vi "Set FPGA constants.vi"(8 "error in (no error)":errorcluster, 11 "AODAcq in":refnum<class "AODAcq.lvclass">) -> (0 "error out":errorcluster, 3 "AODAcq out":refnum<class "AODAcq.lvclass">)   [LabVIEW 2011, in "AODAcq.lvclass"]
uses:
  AODAcq.lvclass
  FPGA_Control/AODCalibration.ctl
  <vilib>/Utility/error.llb/Error Cluster From Error Code.vi
  Program Files/National Instruments/LabVIEW 2011/Targets/NI/FPGA/StockFPGA_IntfPrivate/ScriptTemplates/StockFPGA_PlugInRead32.vi
  <vilib>/rvi/errors/niLvFpgaAdjustHostInterfaceError.vi
  <vilib>/rvi/interface/nirviReadWriteControl/nirviReadWriteControl.xnode
  FPGA_Control/AODRef.ctl
  FPGA Bitfiles/Acquisition_FPGATarget_AODControl(FPGA)_C1C38267.lvbitx
  FPGA_Control/AOD Control (FPGA).vi
  NiFpgaLv.dll
  <vilib>/FPGAPlugInAG/PXIe-7965R/niLvFpga_Read32_PXIe-7965R.vi
  <vilib>/rvi/interface/nirviReadWriteControl/niFpgaRWControlAccessTimeoutTemplate.vi
panel:
  in  "AOD.BlankSamples":u16=800
  in  "AOD.ThrowawaySamples":u16=1250
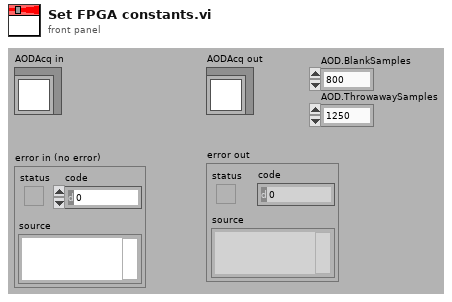
[diagram p1: front panel]
types:
  T1 = typedef "AODCalibration.ctl" = cluster{"XHP ChirpGain":fxp<+/-,16,2>, "YHP ChirpGain":fxp<+/-,16,2>, "XLP ChirpGain":fxp<+/-,16,2>, "YLP ChirpGain":fxp<+/-,16,2>}
  T2 = typedef "AODRef.ctl" = refnum<k20>
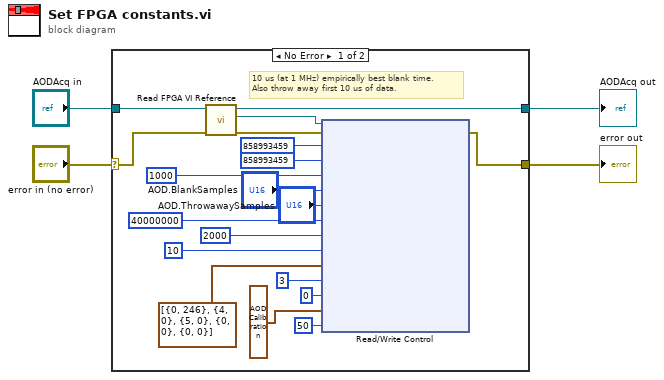
[diagram p0: block diagram]
diagram:
  n1 = case shown="No Error" "error in (no error)" {
    selector: "error in (no error)" -> [w15 w25]
    tunnel: [w14 w25] -> w3
    tunnel: [w22 w24] -> w1
    tunnel: "AODAcq in" -> [w23 w24]
    frame No Error {
      # "10 us (at 1 MHz) empirically best blank time.\nAlso throw away first 10 us of data."
      n2 = call-dynamic "Read FPGA VI Reference.vi"("error in (no error)"=w15, "AODAcq in"=w23) -> ("error out"=w20:errorcluster, "FPGA VI Reference"=w21:T2, "AODAcq out"=w22:refnum<class "AODAcq.lvclass">)  [unwired: 7 in]
      n3 = xnode "Read/Write Control"("FPGA VI Reference In"=w21, "error in"=w20, "AOD.HP Center Frequency"=u32 858993459 ("LP Center Frequency"), "AOD.LP Center Frequency"=u32 858993459 ("LP Center Frequency"), "Setup.Downsample"=u32 1000 ("Downsample"), "AOD.BlankSamples"="AOD.BlankSamples", "AOD.ThrowawaySamples"="AOD.ThrowawaySamples", "Update IO timeout"=u32 40000000 ("Setup.PMT Timeout"), "AOD.UpdatesPerPoint"=u32 2000, "Comm.P high"=u32 10 ("P high"), "Debug.FinishedSetting"=cluster{"Address":u8, "Value":u32}[] [{"Address"=0, "Value"=246}, {"Address"=4, "Value"=0}, {"Address"=5, "Value"=0}, {"Address"=0, "Value"=0}, {"Address"=0, "Value"=0}], "Debug.FinishedSettingSize"=i16 3, "Setup.BitShift"=i16 0, "AOD.Calibration"=T1 {"XHP ChirpGain"=1.0, "YHP ChirpGain"=1.0, "XLP ChirpGain"=1.0, "YLP ChirpGain"=1.0}, "Comm.UpdateIO time"=u32 50) -> ("error out"=w14:errorcluster)  [unwired: 1 out]
    }
    frame Error {
    }
  }
  "error out" <- w3
  "AODAcq out" <- w1
